vi "Inputs_DriverStation.vi"() -> ()   [LabVIEW 2018]
panel:
  out "Super_Test_Mode":bool=TRUE
  out "J1-LeftJoystickButton":bool
  out "Tune_Tab":bool
  out "J1-RightJoystickButton":bool
  out "J1-LeftBumper":bool
  out "J1-RightBumper":bool
  out "J1-Menu":bool
  out "Elevator_Kf_Climb":dbl
  out "J1-View":bool
  out "Climb_Level":bool
  out "Master_Safety_Override":bool
  out "DS Elevator Buttons":T1
  out "Drive_Encoder_Reset":bool
  out "Vacuum_Pump":dbl
  out "Elevator_Kf_3":dbl
  out "Elevator_Kf_2":dbl
  out "Elevator_Manual":bool=TRUE
  out "J1-RightX":dbl=0.015748031496062992
  out "J1-LeftY":dbl=0.05511811023622047
  out "J1-LeftTrigger":dbl
  out "J1-RightTrigger":dbl
  out "J1-Y":bool
  out "J1-X":bool
  out "J1-B":bool
  out "J1-A":bool
  out "J1-DPAD":i16=-1
  out "Elevator_Kf_1":dbl
  out "Y Joystick":dbl
  out "X Joystick":dbl
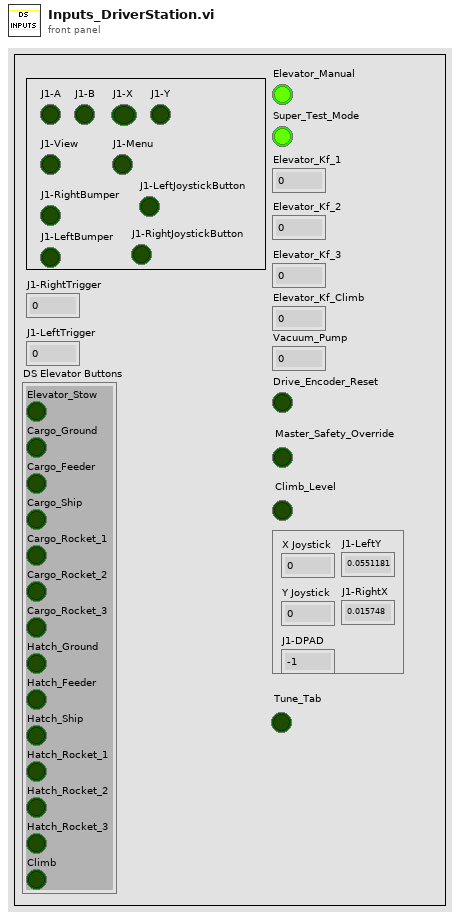
[diagram p1: front panel]
types:
  T1 = cluster{"Elevator_Stow":bool, "Cargo_Ground":bool, "Cargo_Feeder":bool, "Cargo_Ship":bool, "Cargo_Rocket_1":bool, "Cargo_Rocket_2":bool, "Cargo_Rocket_3":bool, "Hatch_Ground":bool, "Hatch_Feeder":bool, "Hatch_Ship":bool, "Hatch_Rocket_1":bool, "Hatch_Rocket_2":bool, "Hatch_Rocket_3":bool, "Climb":bool}
diagram:
